vi "ReadPositionFromAxis.vi"(8 "error in (no error)":errorcluster, 11 "Picomotor8742 in":refnum<class "Picomotor8742.lvclass">) -> (0 "error out":errorcluster, 3 "Picomotor8742 out":refnum<class "Picomotor8742.lvclass">)   [LabVIEW 2020, in "Picomotor8742.lvclass"]
doc: "Read the axis positions from the physical device and write it to the CVT"
uses:
  Picomotor8742.lvclass
  Picomotor8742.lvclass/Picomotor8742.ctl
  Picomoto8742ControllerClass.lvclass
panel:
  out "total time":u32
  out "read position time":u32
  out "time for add to cvt and settings cluster":u32
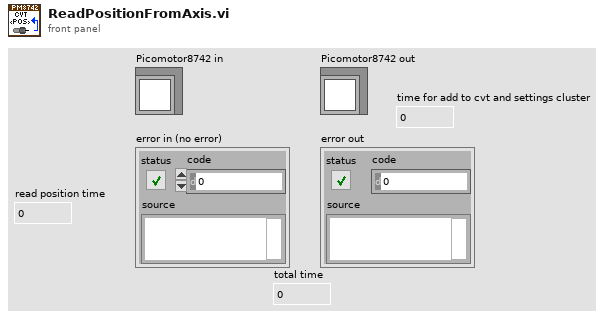
[diagram p1: front panel]
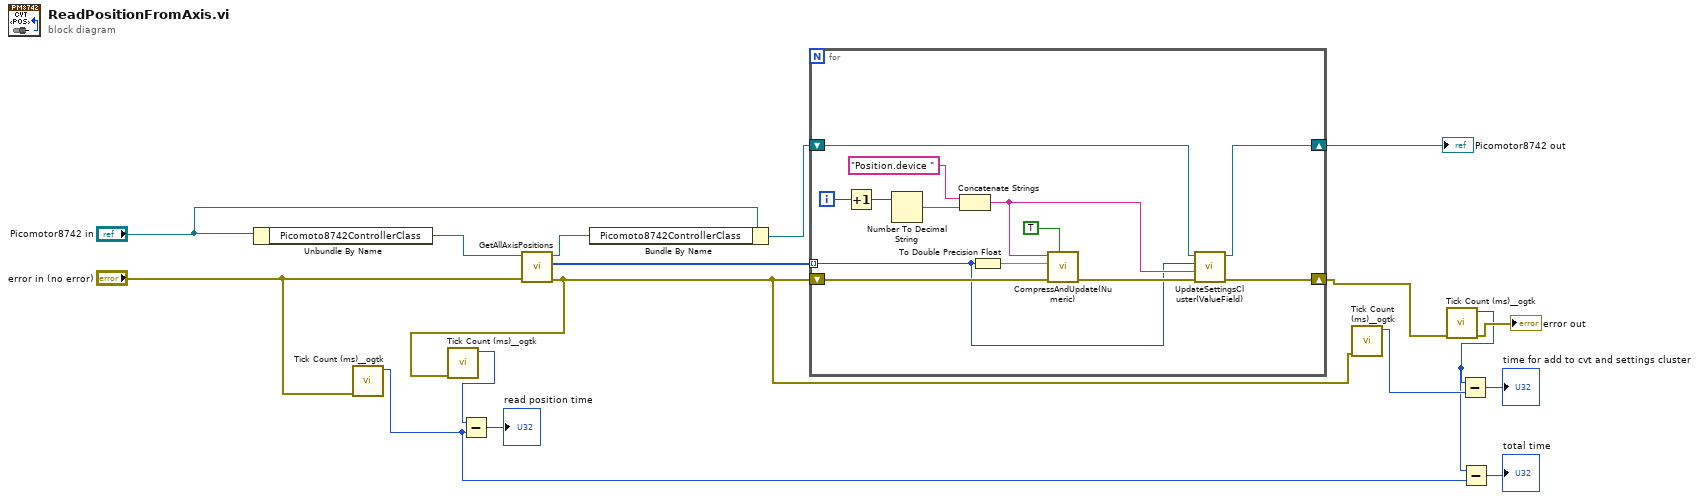
[diagram p0: block diagram]
diagram:
  n1 = Unbundle By Name("Picomotor8742 in") -> ("Picomoto8742ControllerClass"=w16:refnum<class "Picomoto8742ControllerClass.lvclass">)
  n2 = call "Tick Count (ms)__ogtk.vi"("error in (no error)"="error in (no error)") -> ("millisecond timer value"=w2:u32)  [unwired: 9 in, 1 out]
  n3 = call "Tick Count (ms)__ogtk.vi"("error in (no error)"="error in (no error)") -> ("millisecond timer value"=w5:u32)  [unwired: 9 in, 1 out]
  n4 = Subtract(x=w5, y=w2) -> (x-y=→"read position time":u32)
  n5 = call-dynamic "GetAllAxisPositions.vi"("error in (no error)"="error in (no error)", "Picomoto8742ControllerClass in"=w16) -> ("error out"=w11:errorcluster, "AxisPositions"=w17:i32[], "Picomoto8742ControllerClass out"=w15:refnum<class "Picomoto8742ControllerClass.lvclass">)  [unwired: 7 in]
  n6 = Bundle By Name(cluster="Picomotor8742 in", "Picomoto8742ControllerClass"=w15) -> (w14:refnum<class "Picomotor8742.lvclass">)
  n7 = for {
    tunnel: w17 -> [w18] mode=indexing
    shift-right: [w22] -> w10
    shift-left: w11 -> [w26]
    shift-right: [w19] -> w12
    shift-left: w14 -> [w20]
    i -> [w30]
    n8 = Increment(x=w30) -> (x+1=w29:i32)
    n9 = Number To Decimal String(number=w29) -> (decimal integer string=w28:string)  [unwired: 1 in]
    n10 = Concatenate Strings("Position.device ", w28) -> (w21:string)
    n11 = To Double Precision Float(number=w18) -> (double precision float=w24:dbl)
    n12 = call "CompressAndUpdate(Numeric).vi"("force CVT update (false)"=TRUE, "error in"=w26, "Numeric"=w24, "command or variable name"=w21) -> ("error out"=w23:errorcluster)  [unwired: 7 in]
    n13 = call-dynamic "UpdateSettingsCluster(ValueField).vi"("error in (no error)"=w23, "SubClusterName"=w21, "Value"=w18, "Picomotor8742 in"=w20) -> ("error out"=w22:errorcluster, "Picomotor8742 out"=w19:refnum<class "Picomotor8742.lvclass">)  [unwired: 6 in]
  }
  "Picomotor8742 out" <- w12
  n14 = call "Tick Count (ms)__ogtk.vi"("error in (no error)"=w11) -> ("millisecond timer value"=w8:u32)  [unwired: 9 in, 1 out]
  n15 = call "Tick Count (ms)__ogtk.vi"("error in (no error)"=w10) -> ("error out"=→"error out":errorcluster, "millisecond timer value"=w3:u32)  [unwired: 9 in]
  n16 = Subtract(x=w3, y=w8) -> (x-y=→"time for add to cvt and settings cluster":u32)
  n17 = Subtract(x=w3, y=w2) -> (x-y=→"total time":u32)
